vi "Host - TX data interpolation test.vi"() -> ()   [LabVIEW 2019]
uses:
  <vilib>/Analysis/1siggen.llb/Ramp Pattern by Samples.vi
  6133229a-d82c-48cf-81c4-6bc8cbbef8c2.vi
  <vilib>/rvi/interface/RandomDataEmulation/nirviRandomDataOpen.vi
  <vilib>/rvi/interface/common/niFpgaCacheSessionInfoDynamic.vi
  <vilib>/Utility/error.llb/Error Cluster From Error Code.vi
  <vilib>/rvi/errors/niLvFpgaAdjustHostInterfaceError.vi
  <vilib>/rvi/interface/common/niFpgaWaitOnOcc.vi
  <vilib>/FPGAPlugInAG/Dynamic/niLvFpga_Close_Dynamic.vi
  <vilib>/rvi/interface/nirviOpenFPGA/nirviOpenFPGA.xnode
  FPGA/Test/TX data interpolation test.vi
  <vilib>/rvi/interface/nirviReadWriteControl/nirviReadWriteControl.xnode
  <vilib>/rvi/interface/nirviMethod/nirviMethod.xnode
  <vilib>/rvi/interface/nirviCloseFPGA/nirviCloseFPGA.xnode
  <vilib>/Analysis/NI_AALBase.lvlib
  <vilib>/FPGAPlugInAG/Dynamic/niLvFpga_WriteFifo_Dynamic.vi
  <vilib>/rvi/errors/niLvFpgaMergeErrorWithErrorCode.vi
  NiFpgaLv.dll
  <vilib>/rvi/interface/Simulation/niFpgaSimulationCallBeginRW.vi
  <vilib>/FPGAPlugInAG/Dynamic/niLvFpga_ConfigureFifo_Dynamic.vi
  <vilib>/FPGAPlugInAG/Dynamic/niLvFpga_ReadFifo_Dynamic.vi
panel:
  out "Plot":waveform(dbl)[](graph)
  in  "fetch":bool
  out "samples interpolated":u32
  out "status":string
  out "Elements Remaining":u32
  in  "stop":bool
  in  "input sample rate":fxp<+,48,1>=0.10000000000000142
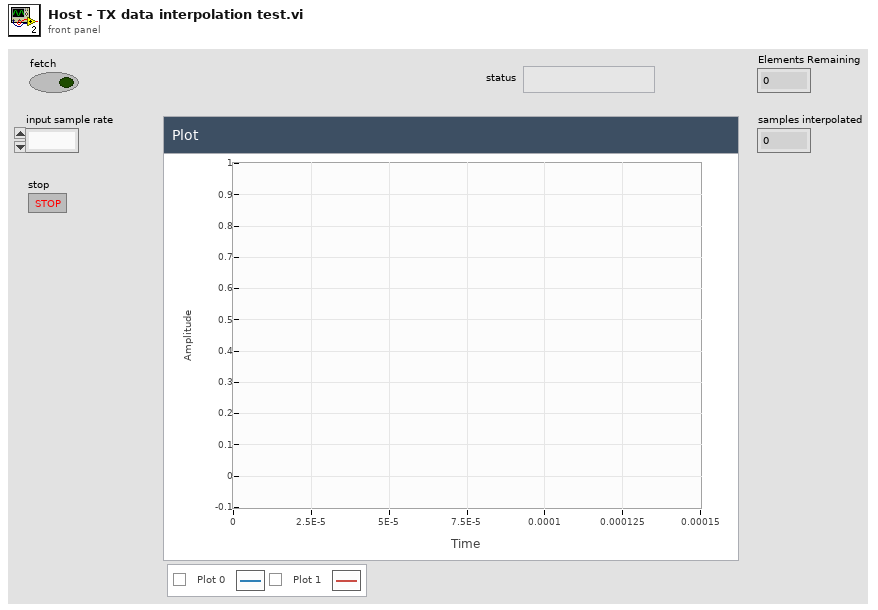
[diagram p1: front panel]
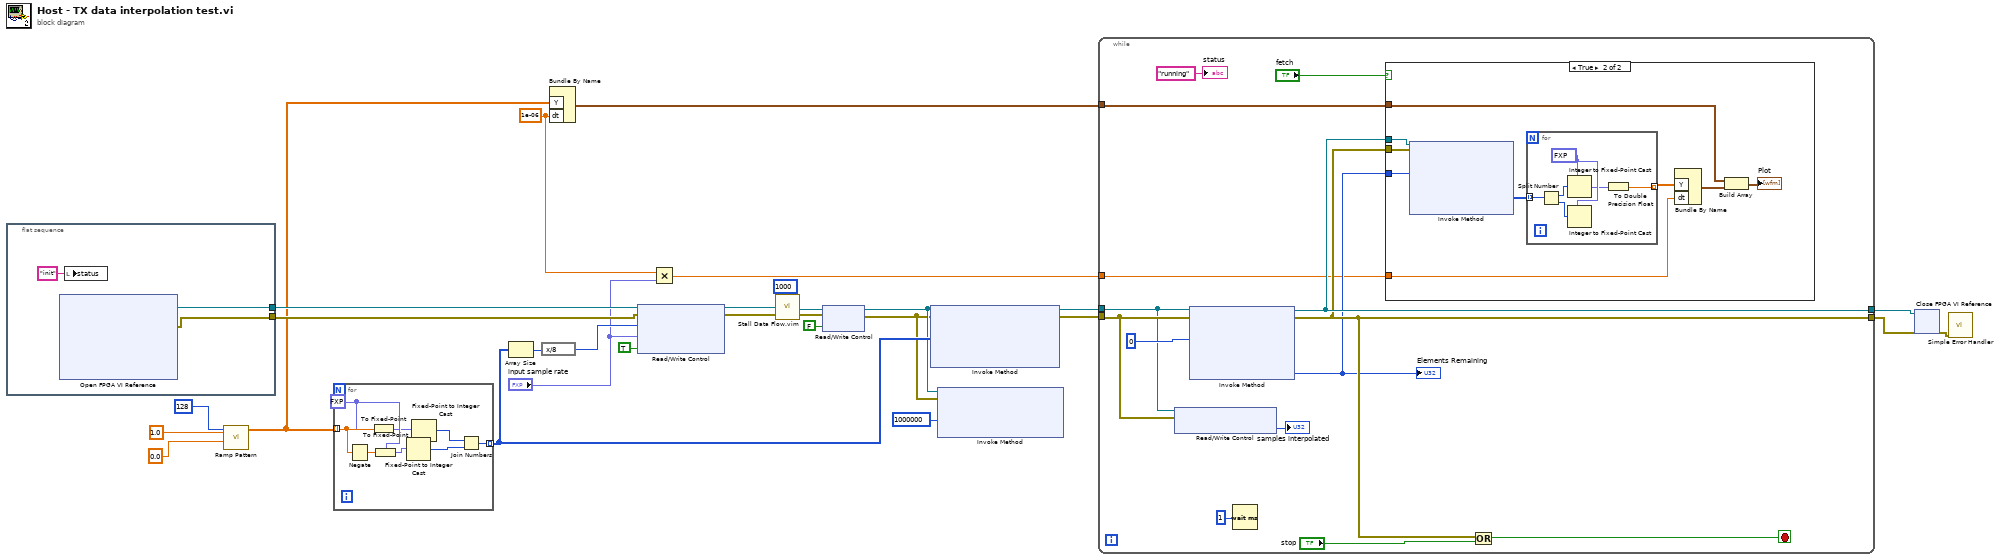
[diagram p0: block diagram]
diagram:
  w3 = 1e-06 ("dt")
  n1 = flat-sequence {
    tunnel: [w30] -> w27
    tunnel: [w29] -> w21
    frame #0 {
      n2 = xnode "Open FPGA VI Reference"() -> ("FPGA VI Reference Out"=w30:refnum<k20>, "error out"=w29:errorcluster)  [unwired: 2 in]
      n3 = local write "status"("init" ("status")) -> ()
    }
  }
  n4 = call-poly <vilib>:"Ramp Pattern.vi"("start"=0.0 ("end"), "end"=1.0, "samples"=128) -> ("Ramp Pattern"=w5:dbl[])  [unwired: 7 in, 1 out]
  n5 = for {
    tunnel: w5 -> [w38] mode=indexing
    tunnel: [w31] -> w14 mode=indexing
    w36 = fxp<+/-,16,1> 0.0 ("fixed-point type")
    n6 = Negate(x=w38) -> (-x=w37:dbl)
    n7 = To Fixed-Point(fixed-point type=w36, number=w38) -> (fixed-point=w35:fxp<+/-,16,1>)
    n8 = To Fixed-Point(fixed-point type=w36, number=w37) -> (fixed-point=w34:fxp<+/-,16,1>)
    n9 = Fixed-Point to Integer Cast(1:w34) -> (0:w33:i16)
    n10 = Fixed-Point to Integer Cast(1:w35) -> (0:w32:i16)
    n11 = Join Numbers(hi=w32, lo=w33) -> ((hi.lo)=w31:u32)
  }
  n12 = Array Size(array=w14) -> (size(s)=w23:i32)
  n13 = expression code="x/8"(w23) -> (w22:i32)
  n14 = Bundle By Name("Y"=w5, "dt"=w3) -> (w1:waveform(dbl))  [unwired: 1 in]
  n15 = xnode "Read/Write Control"("FPGA VI Reference In"=w27, "error in"=w21, "burst size"=w22, "input sample rate"="input sample rate", "reset"=TRUE) -> ("FPGA VI Reference Out"=w17:refnum<k20>, "error out"=w16:errorcluster)
  n16 = Multiply(x=w3, y="input sample rate") -> (x*y=w2:dbl)
  n17 = call "Stall Data Flow.vim"("value in"=w17, "milliseconds to wait"=u32 1000) -> ("value out"=w18:refnum<k20>)  [unwired: 1 out]
  n18 = xnode "Read/Write Control"("FPGA VI Reference In"=w18, "error in"=w16, "reset"=FALSE) -> ("FPGA VI Reference Out"=w11:refnum<k20>, "error out"=w10:errorcluster)
  n19 = xnode "Invoke Method"("FPGA VI Reference In"=w11, "error in"=w10, "Data"=w14) -> ("FPGA VI Reference Out"=w13:refnum<k20>, "error out"=w12:errorcluster)  [unwired: 1 in, 1 out]
  n20 = xnode "Invoke Method"("FPGA VI Reference In"=w11, "error in"=w10, "Requested Depth"=u32 1000000) -> ()  [unwired: 3 out]
  n21 = while {
    tunnel: w13 -> [w47]
    tunnel: w12 -> [w48]
    tunnel: [w44] -> w8
    tunnel: [w42] -> w7
    tunnel: w2 -> [w40]
    tunnel: w1 -> [w39]
    stop <- w46 stop-if-true
    n22 = xnode "Read/Write Control"("FPGA VI Reference In"=w47, "error in"=w48) -> ("samples interpolated"=→"samples interpolated":u32)  [unwired: 2 out]
    n23 = xnode "Invoke Method"("FPGA VI Reference In"=w47, "error in"=w48, "Number of Elements"=u32 0) -> ("FPGA VI Reference Out"=w44:refnum<k20>, "error out"=w42:errorcluster, "Elements Remaining"=w41:u32)  [unwired: 1 in, 1 out]
    "Elements Remaining" <- w41
    n24 = Wait (ms)(milliseconds to wait=u32 1) -> ()  [unwired: 1 out]
    n25 = case shown="True" "fetch" {
      tunnel: w44 -> [_ w60]
      tunnel: w42 -> [_ w61]
      tunnel: w41 -> [_ w59]
      tunnel: w40 -> [_ w56]
      tunnel: w39 -> [_ w54]
      frame False {
      }
      frame True {
        n26 = xnode "Invoke Method"("FPGA VI Reference In"=w60, "error in"=w61, "Number of Elements"=w59) -> ("Data"=w58:u32[])  [unwired: 1 in, 3 out]
        n27 = for {
          tunnel: w58 -> [w67] mode=indexing
          tunnel: [w62] -> w57 mode=indexing
          w64 = fxp<+/-,16,1> 0.0 ("fixed-point type")
          n28 = Split Number(x=w67) -> (hi(x)=w66:u16, lo(x)=w65:u16)
          n29 = Integer to Fixed-Point Cast(fixed-point type=w64, integer=w66) -> (fixed-point=w63:fxp<+/-,16,1>)
          n30 = Integer to Fixed-Point Cast(fixed-point type=w64, integer=w65) -> ()  [unwired: 1 out]
          n31 = To Double Precision Float(number=w63) -> (double precision float=w62:dbl)
        }
        n32 = Bundle By Name("Y"=w57, "dt"=w56) -> (w55:waveform(dbl))  [unwired: 1 in]
        n33 = Build Array(w54, w55) -> (→"Plot":waveform(dbl)[])
      }
    }
    n34 = Or(x=w42, y="stop") -> (x .or. y?=w46:bool)
    "status" <- "running" ("status")
  }
  n35 = xnode "Close FPGA VI Reference"("FPGA VI Reference In"=w8, "error in"=w7) -> ("error out"=w6:errorcluster)
  n36 = call <vilib>:"Simple Error Handler.vi"("error in (no error)"=w6) -> ()  [unwired: 4 in, 5 out]
